vi "Destroy.vi"(8 "error in (no error)":errorcluster, 11 "timing status pointer":refnum<class "Timing Status.lvclass">) -> (0 "error out":errorcluster)   [LabVIEW 2017, in "DSF Core.lvlib" / "Timing Status.lvclass"]
uses:
  Timing Status.lvclass
  C:/Git/DSF/LabVIEW-Memory/Source/Classes/Pointer/Pointer.lvclass
  LabVIEW-Memory/Source/Classes/Pointer/Pointer.lvclass
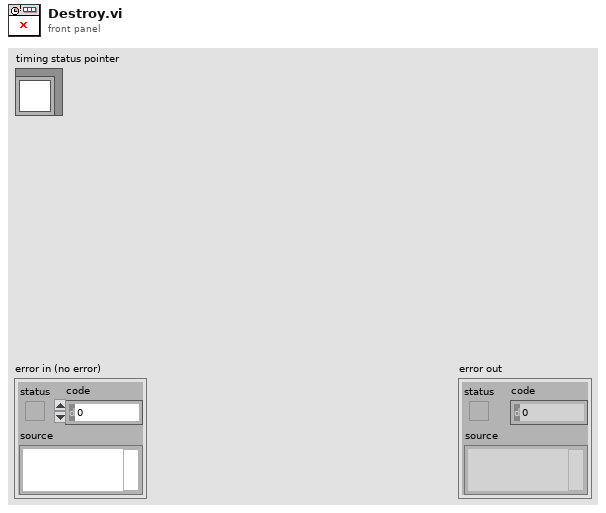
[diagram p1: front panel]
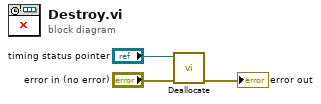
[diagram p0: block diagram]
diagram:
  n1 = call "Deallocate.vi"("error in (no error)"="error in (no error)", "Pointer in"="timing status pointer") -> ("error out"=→"error out":errorcluster)  [unwired: 8 in, 1 out]
